vi "clearpath_initialize_xmitqueue.vi"(1 "Cluster":cluster{i32[], i32, i32}, 2 "Queue Name":string) -> (0 "Xmit Queue":refnum<queue>)   [LabVIEW 2010, in "clearpath_interface.lvlib"]
uses:
  clearpath_interface.lvlib
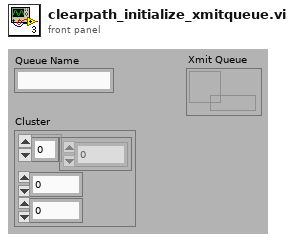
[diagram p1: front panel]
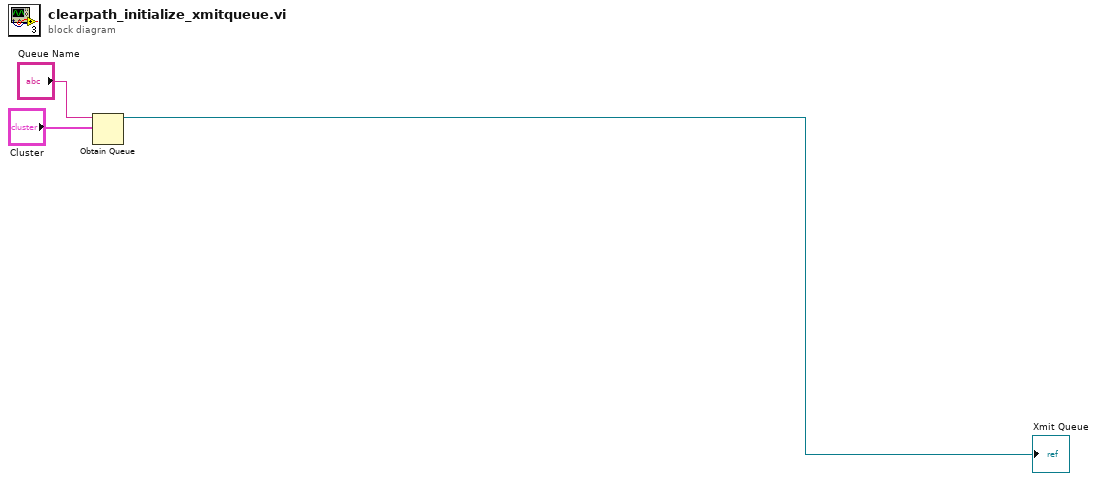
[diagram p0: block diagram]
diagram:
  n1 = Obtain Queue(name (unnamed)="Queue Name", element data type="Cluster") -> (queue out=→"Xmit Queue":refnum<queue>)  [unwired: 3 in, 2 out]
